vi "T_step_PPMS.vi"   [LabVIEW 2019]
uses:
  Global/Global Variables/global.vi
  Instrument_Setup.vi
  Global/Global Variables/Data_Display_global.vi
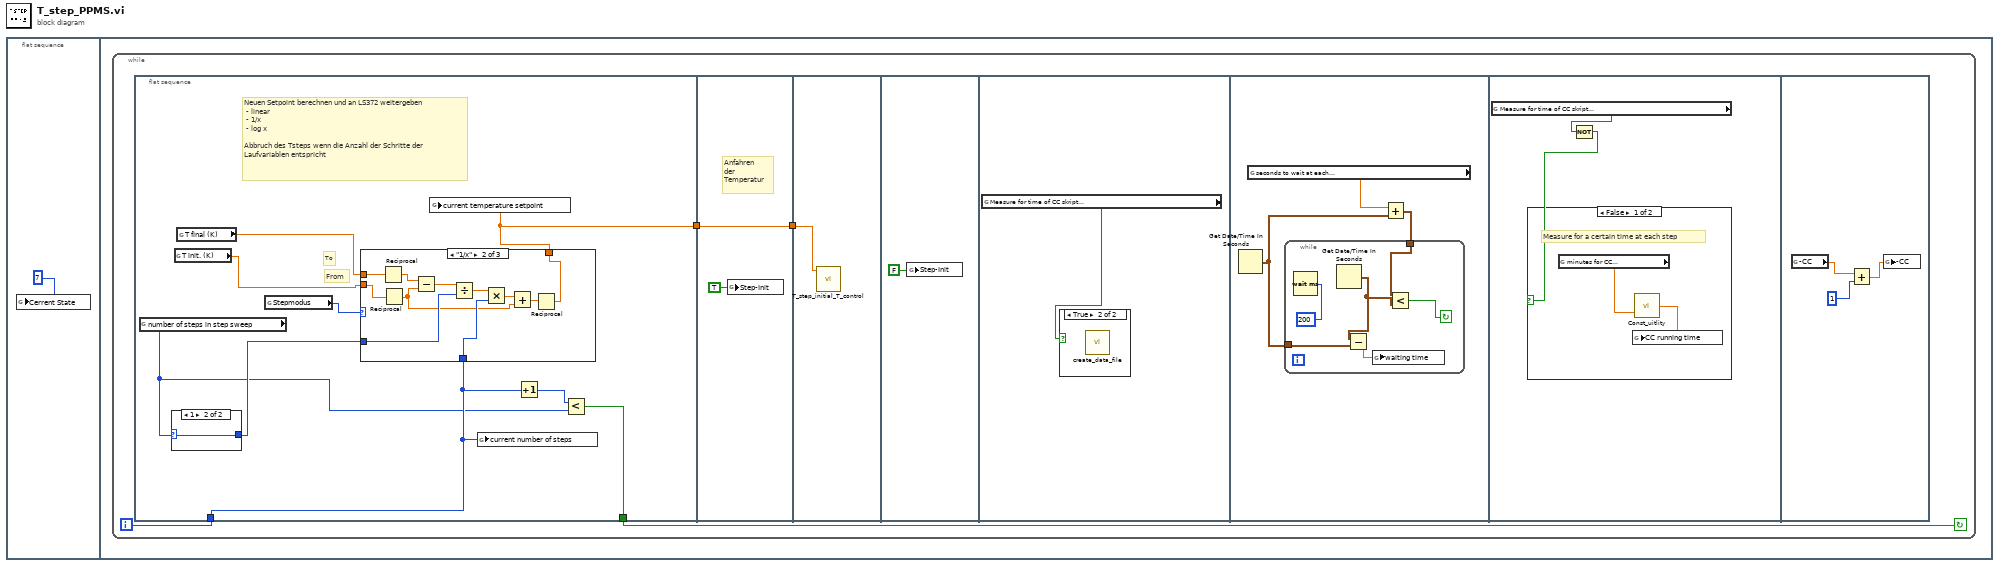
[diagram p0: block diagram]
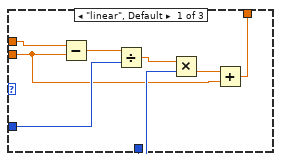
[diagram p2: hidden frame]
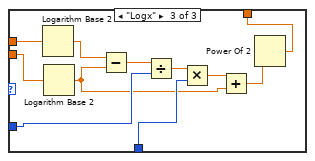
[diagram p3: hidden frame]
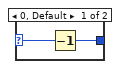
[diagram p4: hidden frame]
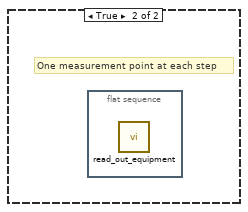
[diagram p6: hidden frame]
diagram:
  n1 = flat-sequence {
    frame #0 {
      n2 = global write "global.vi" "Cerrent State"(7) -> ()
    }
    frame #1 {
      n3 = while {
        i -> [w5]
        stop <- w4 continue-if-true
        n4 = flat-sequence {
          tunnel: w5 -> [w10]
          tunnel: [w7] -> w4
          tunnel: [w6] -> w2
          tunnel: [w48] -> w3
          tunnel: w2 -> [w48]
          tunnel: w3 -> [w50]
          frame #0 {
            # "From"
            # "To"
            # "Neuen Setpoint berechnen und an LS372 weitergeben\n - linear\n - 1/x\n - log x\n\nAbbruch des Tsteps wenn die Anzahl der Schritte der \nLaufvariablen entspricht"
            n5 = global read "global.vi" "number of steps in step sweep"() -> (w8:i32)
            n6 = case shown="1" w8 {
              selector: w8 -> [w46 w47]
              tunnel: [w45 w47] -> w11
              frame 0, Default {
                n7 = Decrement(x=w46) -> (x-1=w45:i32)
              }
              frame 1 {
              }
            }
            n8 = global read "global.vi" "T init. (K)"() -> (w12:dbl)
            n9 = global read "global.vi" "T final (K)"() -> (w13:dbl)
            n10 = global read "Instrument_Setup.vi" "Stepmodus"() -> (w14:enum16{"linear", "1/x", "Logx"})
            n11 = case shown="\"1/x\"" w14 {
              tunnel: w13 -> [w22 w33 w44]
              tunnel: w12 -> [w16 w32 w43]
              tunnel: w11 -> [w20 w29 w40]
              tunnel: w10 -> [w18 w27 w38]
              tunnel: [w15 w23 w34] -> w6
              frame "linear", Default {
                n12 = Subtract(x=w22, y=w16) -> (x-y=w21:dbl)
                n13 = Divide(x=w21, y=w20) -> (x/y=w19:dbl)
                n14 = Multiply(x=w19, y=w18) -> (x*y=w17:dbl)
                n15 = Add(x=w17, y=w16) -> (x+y=w15:dbl)
              }
              frame "1/x" {
                n16 = Reciprocal(x=w33) -> (1/x=w31:dbl)
                n17 = Reciprocal(x=w32) -> (1/x=w25:dbl)
                n18 = Subtract(x=w31, y=w25) -> (x-y=w30:dbl)
                n19 = Divide(x=w30, y=w29) -> (x/y=w28:dbl)
                n20 = Multiply(x=w28, y=w27) -> (x*y=w26:dbl)
                n21 = Add(x=w26, y=w25) -> (x+y=w24:dbl)
                n22 = Reciprocal(x=w24) -> (1/x=w23:dbl)
              }
              frame "Logx" {
                n23 = Logarithm Base 2(1:w44) -> (0:w42:dbl)
                n24 = Logarithm Base 2(1:w43) -> (0:w36:dbl)
                n25 = Subtract(x=w42, y=w36) -> (x-y=w41:dbl)
                n26 = Divide(x=w41, y=w40) -> (x/y=w39:dbl)
                n27 = Multiply(x=w39, y=w38) -> (x*y=w37:dbl)
                n28 = Add(x=w37, y=w36) -> (x+y=w35:dbl)
                n29 = Power Of 2(x=w35) -> (2^x=w34:dbl)
              }
            }
            n30 = global write "Data_Display_global.vi" "current temperature setpoint"(w6) -> ()
            n31 = global write "Data_Display_global.vi" "current number of steps"(w10) -> ()
            n32 = Increment(x=w10) -> (x+1=w9:i32)
            n33 = Less?(x=w9, y=w8) -> (x < y?=w7:bool)
          }
          frame #1 {
            # "Anfahren \nder \nTemperatur"
            n34 = global write "global.vi" "Step-Init"(TRUE) -> ()
          }
          frame #2 {
            n35 = call "T_step_initial_T_control.vi"("Current T step Setpoint"=w50) -> ()  [unwired: 11 in]
          }
          frame #3 {
            n36 = global write "global.vi" "Step-Init"(FALSE) -> ()
          }
          frame #4 {
            n37 = global read "Instrument_Setup.vi" "Measure for time of CC skript\nat each field step point"() -> (w52:bool)
            n38 = case shown="True" w52 {
              frame False {
              }
              frame True {
                n39 = call "create_data_file.vi"() -> ()  [unwired: 3 in]
              }
            }
          }
          frame #5 {
            n40 = Get Date/Time In Seconds() -> (seconds since 1Jan1904=w53:timestamp)
            n41 = global read "Instrument_Setup.vi" "seconds to wait at each\nfield step in a step sweep"() -> (w55:dbl)
            n42 = Add(x=w55, y=w53) -> (x+y=w54:timestamp)
            n43 = while {
              tunnel: w54 -> [w57]
              tunnel: w53 -> [w60]
              stop <- w56 continue-if-true
              n44 = Wait (ms)(milliseconds to wait=200) -> ()  [unwired: 1 out]
              n45 = Get Date/Time In Seconds() -> (seconds since 1Jan1904=w58:timestamp)
              n46 = Subtract(x=w58, y=w60) -> (x-y=w59:dbl)
              n47 = global write "Data_Display_global.vi" "waiting time"(w59) -> ()
              n48 = Less?(x=w58, y=w57) -> (x < y?=w56:bool)
            }
          }
          frame #6 {
            n49 = global read "Instrument_Setup.vi" "Measure for time of CC skript\nat each field step point"() -> (w63:bool)
            n50 = Not(x=w63) -> (.not. x?=w62:bool)
            n51 = case shown="False" w62 {
              frame False {
                # "Measure for a certain time at each step"
                n52 = global read "Instrument_Setup.vi" "minutes for CC\nto run"() -> (w65:dbl)
                n53 = call "Const_uitlity.vi"("Duration"=w65) -> ("Minutes passed"=w64:dbl)  [unwired: 1 in]
                n54 = global write "Data_Display_global.vi" "CC running time"(w64) -> ()
              }
              frame True {
                # "One measurement point at each step"
                n55 = flat-sequence {
                  frame #0 {
                    n56 = call "read_out_equipment.vi"() -> ()  [unwired: 1 in]
                  }
                }
              }
            }
          }
          frame #7 {
            n57 = global read "global.vi" "-CC"() -> (w68:dbl)
            n58 = Add(x=w68, y=1) -> (x+y=w66:dbl)
            n59 = global write "global.vi" "-CC"(w66) -> ()
          }
        }
      }
    }
  }
